vi "Main_maszyna.vi"() -> ()   [LabVIEW 2013]
doc: "Use this template to build a standard state machine design pattern. Each state executes code and determines which state to transition to. Contrast this design pattern with the User Interface Event Handler pattern, in which code executes in response to user actions. Contrast this design pattern also with the Queued Message Handler pattern, in which each message handling code can queue zero or more new messages.\nNote: This template does not contain the most recent programming guidelines recommended by National Instruments. For a complete, project-based implementation of the Standard State Machine pattern, use the Create Project dialog box instead of this template."
uses:
  inne pliki/Stany.ctl
  inne pliki/Params.ctl
  inne pliki/Data.ctl
  inne pliki/Akcje czas FVG.ctl
panel:
  out "Czas do końca pomiaru":dbl
  in  "bStopPomiar":bool
  out "Warning text":string
  out "Warning":bool
  in  "Temp limits":T1={"Max (25)"=22.0, "Min (0)"=0.0}
  out "Waveform Chart":cluster{"Temperatura":dbl, "Średnia":dbl}(graph)
  in  "Akcje":T2
  out "Stan aktualny":T3
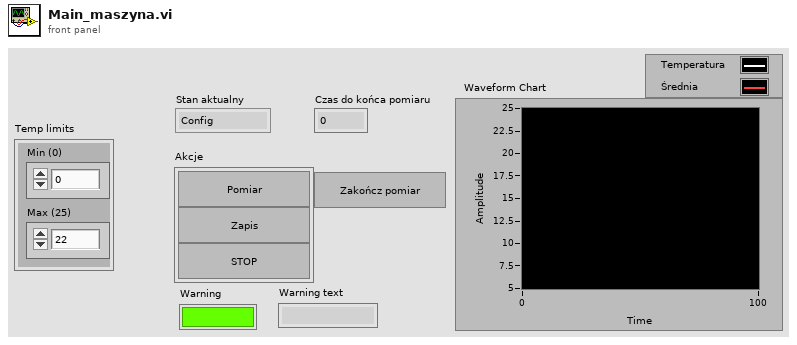
[diagram p1: front panel]
types:
  T1 = typedef "Params.ctl" = cluster{"Max (25)":dbl, "Min (0)":dbl}
  T2 = cluster{"bPomiar":bool, "bZapis":bool, "bSTOP":bool}
  T3 = typedef "Stany.ctl" = enum16{"Config", "IDLE", "Measure", "Analyze", "Display", "STOP", "Save"}
  T4 = typedef "Data.ctl" = cluster{"Temperatura":dbl, "Średnia":dbl, "Warning":bool, "Warning text ":string, "Temp limits":T1, "Temp Array":dbl[], "Sternia Array":dbl[]}
  T5 = typedef "Akcje czas FVG.ctl" = enum16{"Reset", "Wait"}
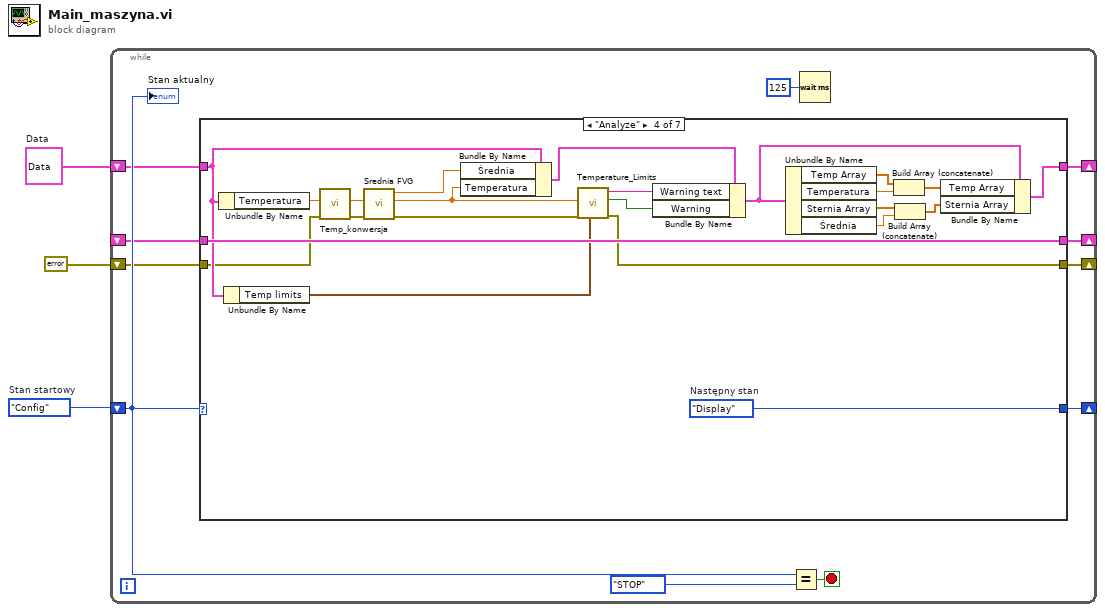
[diagram p0: block diagram]
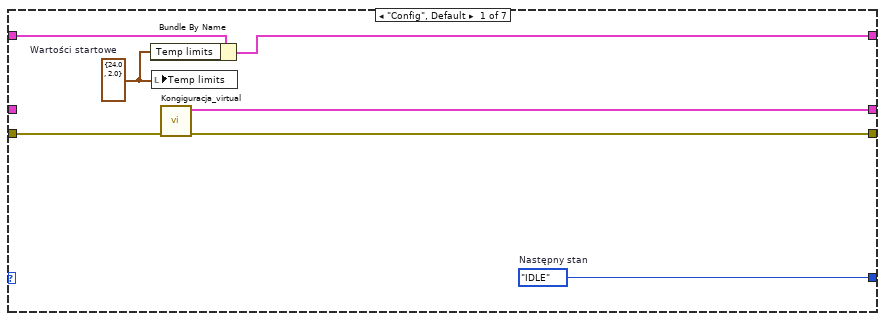
[diagram p2: hidden frame]
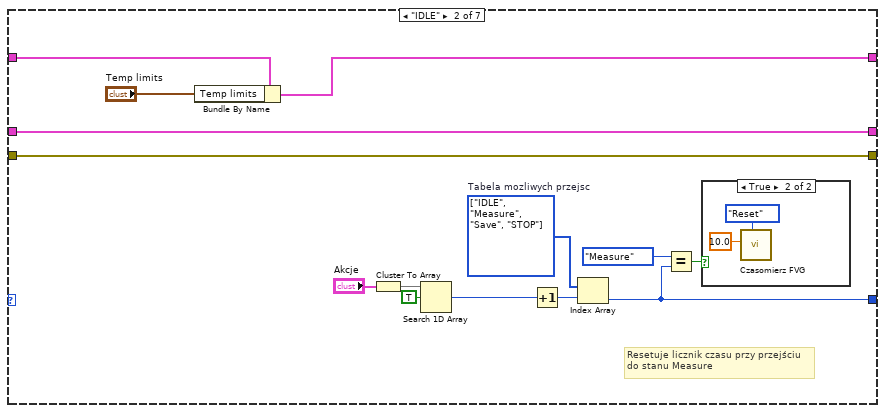
[diagram p3: hidden frame]
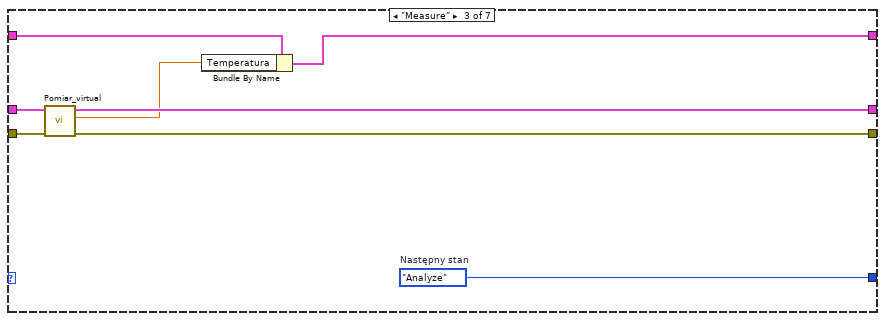
[diagram p5: hidden frame]
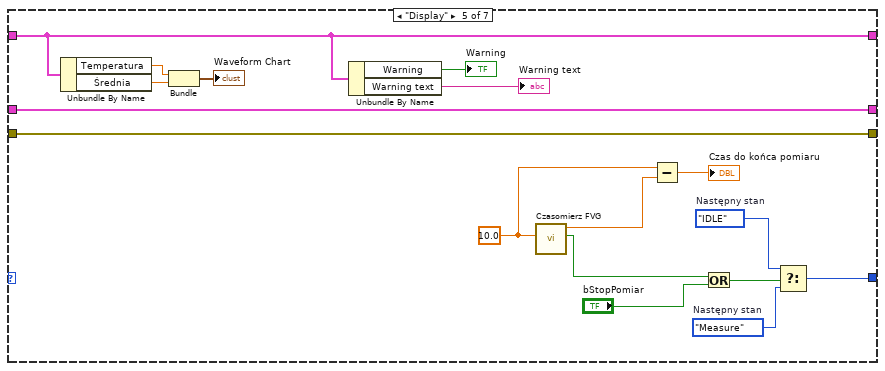
[diagram p6: hidden frame]
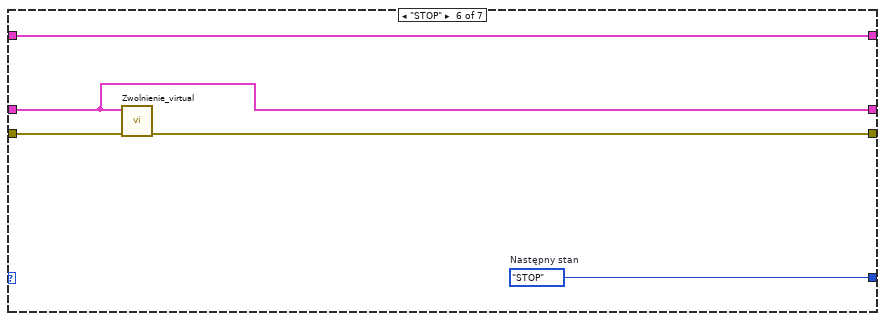
[diagram p7: hidden frame]
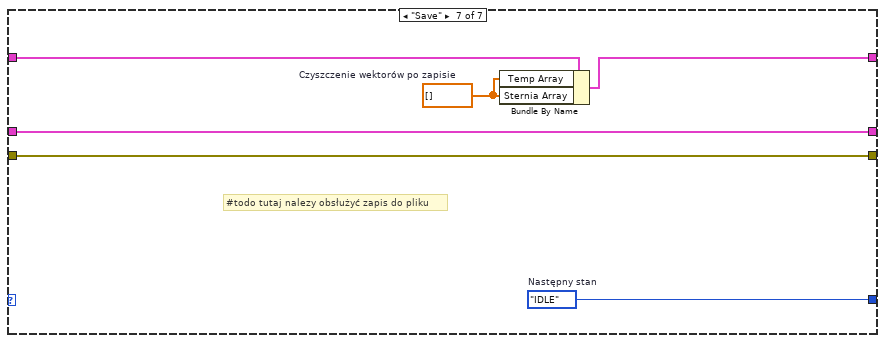
[diagram p8: hidden frame]
diagram:
  w2 = T4 {"Temperatura"=0.0, "Średnia"=0.0, "Warning"=FALSE, "Warning text "="", "Temp limits"={"Max (25)"=25.0, "Min (0)"=0.0}, "Temp Array"=[], "Sternia Array"=[]}  # Data
  w3 = Stany."Config"  # Stan startowy
  n1 = while {
    shift-right: [w12] -> _
    shift-left: w3 -> [w13]
    shift-right: [w8] -> _
    shift-left: w2 -> [w9]
    shift-right: [w7] -> _
    shift-left: _ -> [w6]
    shift-right: [w5] -> _
    shift-left: errorcluster {"status"=FALSE, "code"=0, "source"=""} ("error out") -> [w4]
    stop <- w14 stop-if-true
    n2 = case shown="\"Analyze\"" w13 {
      tunnel: [w21 w23 w45 w68 w76 w90 w96] -> w12
      tunnel: w9 -> [w17 w26 w39 w64 w80 w89 w93]
      tunnel: [w16 w25 w38 w46 w80 w89 w92] -> w8
      tunnel: [w20 w29 w43 w67 w85 w86 w95] -> w7
      tunnel: w6 -> [_ w29 w44 w67 w85 w86 w95]
      tunnel: [w18 w28 w42 w59 w84 w87 w94] -> w5
      tunnel: w4 -> [w19 w28 w41 w60 w84 w88 w94]
      frame "Config", Default {
        w15 = T1 {"Max (25)"=24.0, "Min (0)"=2.0}  # Wartości startowe
        w21 = Stany."IDLE"  # Następny stan
        n3 = Bundle By Name(cluster=w17, "Temp limits"=w15) -> (w16:T4)
        n4 = local write "Temp limits"(w15) -> ()
        n5 = call "Kongiguracja_virtual.vi"("error in (no error)"=w19) -> ("error out"=w18:errorcluster, "Reference out"=w20:cluster{"Numeric":dbl, "Boolean":bool})  [unwired: 9 in]
      }
      frame "IDLE" {
        w30 = T3[] [enum."IDLE", enum."Measure", enum."Save", enum."STOP"] items=["Config", "IDLE", "Measure", "Analyze", "Display", "STOP", "Save"]  # Tabela mozliwych przejsc
        # "Resetuje licznik czasu przy przejściu\ndo stanu Measure"
        n6 = Bundle By Name(cluster=w26, "Temp limits"="Temp limits") -> (w25:T4)
        n7 = Cluster To Array(cluster="Akcje") -> (array=w34:bool[])
        n8 = Search 1D Array(1D array=w34, element=TRUE) -> (index of element=w32:i32)  [unwired: 1 in]
        n9 = Increment(x=w32) -> (x+1=w31:i32)
        n10 = Index Array(array=w30, index=w31) -> (element=w23:T3)
        n11 = Equal?(x=Stany."Measure" ("Następny stan"), y=w23) -> (x = y?=w24:bool)
        n12 = case shown="True" w24 {
          frame False {
          }
          frame True {
            n13 = call "Czasomierz FVG.vi"("Akcja (Wait)"=Akcje_czas_FVG."Reset", "Czas (s)"=10.0) -> ()  [unwired: 7 in, 3 out]
          }
        }
      }
      frame "Measure" {
        w45 = Stany."Analyze"  # Następny stan
        n14 = call "Pomiar_virtual.vi"("error in (no error)"=w41, "Reference in"=w44) -> ("error out"=w42:errorcluster, "out"=w40:dbl, "Reference out"=w43:cluster{"Numeric":dbl, "Boolean":bool})  [unwired: 7 in]
        n15 = Bundle By Name(cluster=w39, "Temperatura"=w40) -> (w38:T4)
      }
      frame "Analyze" {
        w68 = Stany."Display"  # Następny stan
        n16 = Unbundle By Name(w64) -> ("Temperatura"=w66:dbl)
        n17 = Unbundle By Name(w64) -> ("Temp limits"=w65:T1)
        n18 = call "Temp_konwersja.vi"("error in (no error)"=w60, "Temp in"=w66) -> ("error out"=w58:errorcluster, "Temp out"=w57:dbl)  [unwired: 8 in]
        n19 = call "Srednia FVG.vi"("error in (no error)"=w58, "temperatura in"=w57) -> ("error out"=w56:errorcluster, "temperatura out"=w55:dbl, "średnia out"=w54:dbl)  [unwired: 7 in]
        n20 = Bundle By Name(cluster=w64, "Średnia"=w54, "Temperatura"=w55) -> (w61:T4)
        n21 = call "Temperature_Limits.vi"("Temp limits"=w65, "error in (no error)"=w56, "TEMP"=w55) -> ("error out"=w59:errorcluster, "Warning"=w62:bool, "Warning Text"=w63:string)  [unwired: 6 in]
        n22 = Bundle By Name(cluster=w61, "Warning text"=w63, "Warning"=w62) -> (w47:T4)
        n23 = Unbundle By Name(w47) -> ("Temp Array"=w53:dbl[], "Temperatura"=w52:dbl, "Sternia Array"=w51:dbl[], "Średnia"=w50:dbl)
        n24 = Build Array (concatenate)(w53, w52) -> (w49:dbl[])
        n25 = Build Array (concatenate)(w51, w50) -> (w48:dbl[])
        n26 = Bundle By Name(cluster=w47, "Temp Array"=w49, "Sternia Array"=w48) -> (w46:T4)
      }
      frame "Display" {
        w71 = 10.0 ("Czas (s)")
        w75 = Stany."Measure"  # Następny stan
        w77 = Stany."IDLE"  # Następny stan
        n27 = Unbundle By Name(w80) -> ("Temperatura"=w82:dbl, "Średnia"=w83:dbl)
        n28 = Bundle("Temperatura"=w82, "Średnia"=w83) -> (→"Waveform Chart":cluster{"Temperatura":dbl, "Średnia":dbl})  [unwired: 1 in]
        n29 = Unbundle By Name(w80) -> ("Warning"=→"Warning":bool, "Warning text"=→"Warning text":string)
        n30 = call "Czasomierz FVG.vi"("Czas (s)"=w71) -> ("Elapsed?"=w72:bool, "Elapsed Time"=w70:dbl)  [unwired: 8 in, 1 out]
        n31 = Subtract(x=w71, y=w70) -> (x-y=→"Czas do końca pomiaru":dbl)
        n32 = Or(x=w72, y="bStopPomiar") -> (x .or. y?=w74:bool)
        n33 = Select(t=w77, s=w74, f=w75) -> (s? t:f=w76:T3)
      }
      frame "STOP" {
        w90 = Stany."STOP"  # Następny stan
        n34 = call "Zwolnienie_virtual.vi"("error in (no error)"=w88, "Reference in"=w86) -> ("error out"=w87:errorcluster)  [unwired: 9 in]
      }
      frame "Save" {
        w91 = dbl[] []  # Czyszczenie wektorów po zapisie
        w96 = Stany."IDLE"  # Następny stan
        # "#todo tutaj nalezy obsłużyć zapis do pliku"
        n35 = Bundle By Name(cluster=w93, "Temp Array"=w91, "Sternia Array"=w91) -> (w92:T4)
      }
    }
    n36 = Equal?(x=w13, y=Stany."STOP" ("Stan startowy")) -> (x = y?=w14:bool)
    n37 = Wait (ms)(milliseconds to wait=u32 125) -> ()  [unwired: 1 out]
    "Stan aktualny" <- w13
  }
